vi "Get Ramping Mode.vi"(0 "Communications Config":T1={"GPIB address"=22, "GPIB bus"=0, "connection ID"=refnum, "IP"="192.168.2.200", "Active Comm Interface"=0, "Serial Port"="", "Programmer Type"=0} {"Programmer Type" items=["Model 430", "Model 420"]; "Active Comm Interface" items=["TCP/IP (Model 430 Only)", "RS232", "IEEE488"]}, 1 "error in":T2) -> (2 "Ramping Mode":T3(ring)=enum."RAMPING", 3 "Ramping Mode String":string, 4 "error out":T2)   [LabVIEW 2018]
panel:
  in  "GPIB Address":cluster{"GPIB address":i16, "GPIB bus":i16}={"GPIB address"=22, "GPIB bus"=0}
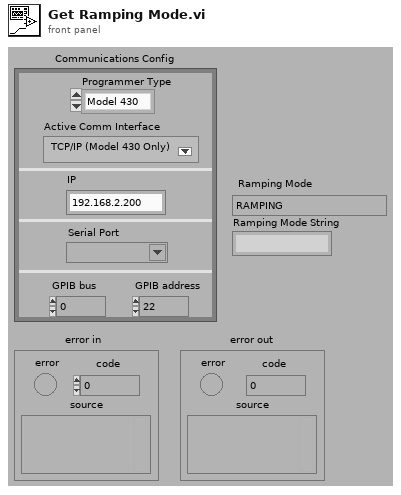
[diagram p1: front panel]
types:
  T1 = cluster{"GPIB address":i16, "GPIB bus":i16, "connection ID":refnum<k5>, "IP":string, "Active Comm Interface":u16, "Serial Port":refnum<visa-resource-name>, "Programmer Type":u16}
  T2 = cluster{"error":bool, "code":i32, "source":string}
  T3 = enum16{"", "RAMPING", "HOLDING", "PAUSED", "MANUAL UP", "MANUAL DOWN", "ZEROING CURRENT", "QUENCH DETECTED", "HEATING SWITCH", "AT ZER0", "COOLING SWITCH"}
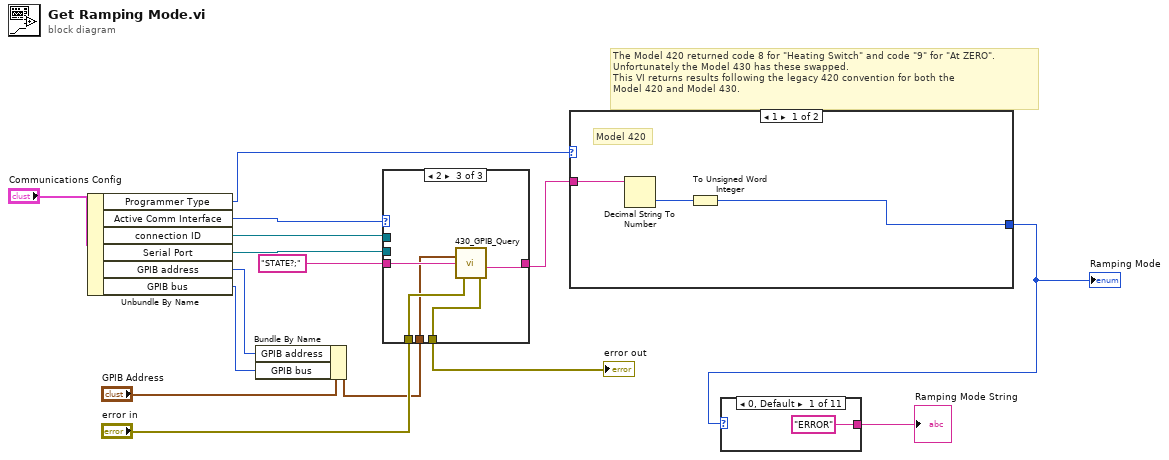
[diagram p0: block diagram]
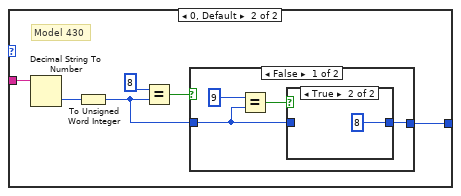
[diagram p2: hidden frame]
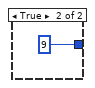
[diagram p4: hidden frame]
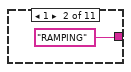
[diagram p5: hidden frame]
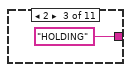
[diagram p6: hidden frame]
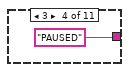
[diagram p7: hidden frame]
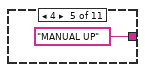
[diagram p8: hidden frame]
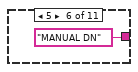
[diagram p9: hidden frame]
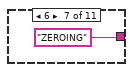
[diagram p10: hidden frame]
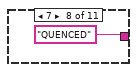
[diagram p11: hidden frame]
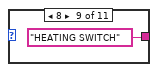
[diagram p12: hidden frame]
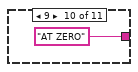
[diagram p13: hidden frame]
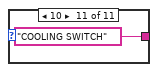
[diagram p14: hidden frame]
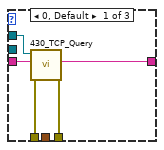
[diagram p15: hidden frame]
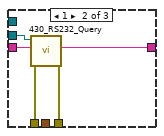
[diagram p16: hidden frame]
diagram:
  # "The Model 420 returned code 8 for \"Heating Switch\" and code \"9\" for \"At ZERO\".\nUnfortunately the Model 430 has these swapped.\nThis VI returns results following the legacy 420 convention for both the\nModel 420 and Model 430."
  n1 = Unbundle By Name("Communications Config") -> ("Programmer Type"=w3:u16, "Active Comm Interface"=w7:u16, "connection ID"=w6:refnum<k5>, "Serial Port"=w5:refnum<visa-resource-name>, "GPIB address"=w8:i16, "GPIB bus"=w9:i16)
  n2 = Bundle By Name(cluster="GPIB Address", "GPIB address"=w8, "GPIB bus"=w9) -> (w11:cluster{"GPIB address":i16, "GPIB bus":i16})
  n3 = case shown="2" w7 {
    tunnel: "STATE?;" -> [w20 w25 w30]
    tunnel: "error in" -> [w19 w24 w29]
    tunnel: [w18 w23 w28] -> w13
    tunnel: w11 -> [_ _ w27]
    tunnel: w6 -> [w17 _ _]
    tunnel: w5 -> [_ w22 _]
    tunnel: [w16 w21 w26] -> w1
    frame 0, Default {
      n4 = call "430_TCP_Query.vi"("error in (no error)"=w19, "Command"=w20, "connection ID"=w17) -> ("error out"=w18:errorcluster, "Response"=w16:string)  [unwired: 4 in, 3 out]
    }
    frame 1 {
      n5 = call "430_RS232_Query.vi"("error in (no error)"=w24, "Command"=w25, "VISA resource name"=w22) -> ("error out"=w23:errorcluster, "Response"=w21:string)  [unwired: 4 in, 3 out]
    }
    frame 2 {
      n6 = call "430_GPIB_Query.vi"("GPIB (In)"=w27, "Input query"=w30, "error in"=w29) -> ("Return string"=w26:string, "error out"=w28:T2)  [unwired: 2 out]
    }
  }
  "error out" <- w13
  n7 = case shown="1" w3 {
    tunnel: [w31 w35] -> w2
    tunnel: w1 -> [w32 w34]
    frame 1 {
      # "Model 420"
      n8 = Decimal String To Number(string=w32) -> (number=w33:i32)  [unwired: 2 in, 1 out]
      n9 = To Unsigned Word Integer(number=w33) -> (unsigned 16bit integer=w31:u16)
    }
    frame 0, Default {
      # "Model 430"
      n10 = Decimal String To Number(string=w34) -> (number=w37:i32)  [unwired: 2 in, 1 out]
      n11 = To Unsigned Word Integer(number=w37) -> (unsigned 16bit integer=w36:u16)
      n12 = Equal?(x=u16 8, y=w36) -> (x = y?=w38:bool)
      n13 = case shown="False" w38 {
        tunnel: w36 -> [w40 _]
        tunnel: [w41 u16 9] -> w35
        frame False {
          n14 = Equal?(x=u16 9, y=w40) -> (x = y?=w42:bool)
          n15 = case shown="True" w42 {
            tunnel: [w44 u16 8] -> w41
            tunnel: w40 -> [w44 _]
            frame False {
            }
            frame True {
            }
          }
        }
        frame True {
        }
      }
    }
  }
  "Ramping Mode" <- w2
  n16 = case shown="0, Default" w2 {
    tunnel: ["ERROR" ("string") "RAMPING" ("string") "HOLDING" ("string") "PAUSED" ("string") "MANUAL UP" ("string") "MANUAL DN" ("string") "ZEROING" ("string") "QUENCED" ("string") "HEATING SWITCH" ("string") "AT ZERO" ("string") "COOLING SWITCH" ("string")] -> w10
    frame 0, Default {
    }
    frame 1 {
    }
    frame 2 {
    }
    frame 3 {
    }
    frame 4 {
    }
    frame 5 {
    }
    frame 6 {
    }
    frame 7 {
    }
    frame 8 {
    }
    frame 9 {
    }
    frame 10 {
    }
  }
  "Ramping Mode String" <- w10
